vi "Amira Bladder Calibration V0.1.vi"() -> ()   [LabVIEW 2020]
uses:
  <userlib>/KQD LabVIEW User/Serial/Controls/SERIAL PortConfig.ctl
  <userlib>/KQD LabVIEW User/Serial/Controls/SERIAL BaudRate.ctl
  <userlib>/Amira UART/Public/TypeDefs/AUART StepDir.ctl
  <vilib>/Utility/file.llb/Write Delimited Spreadsheet (string).vi
  <userlib>/Amira UART/Amira UART.lvclass
  <userlib>/KQD LabVIEW User/Serial/Serial.lvlib
panel:
  out "Data":dbl[][](graph)
  in  "Iteration":i32
  in  "RunWith":cluster{"Steps":i32, "Rates":i32}={"Steps"=400, "Rates"=40}
  in  "Folder":path=path "C:/Amira Data/Strip"
  in  "StartAt":cluster{"Steps":i32, "Rates":i32}={"Steps"=950, "Rates"=200}
  out "Position":dbl[](graph)
  in  "DAQ":tag="Dev1/port0"
  out "UART":string
  in  "ComPort":refnum<visa-resource-name>
  in  "Config":T1={"BaudRate"=enum."460800", "StopBits"=10, "DataBits"=8, "Parity"=enum."None", "FlowControl"=2, "TimeOut"=1000, "TermChar"=10, "ReadTermEn"=TRUE} {"TermChar" format="%.0x"; "FlowControl" items=["None", "XON/XOFF", "RTS/CTS", "XON/XOFF & RTS/CTS", "DTR/DSR", "XON/XOFF & DTR/DSR"]; "DataBits" min=5 max=8 step=1; "StopBits" items=["1.0"=10, "1.5"=15, "2.0"=20]}
  out "ErrOut":errorcluster
  in  "ErrIn":errorcluster
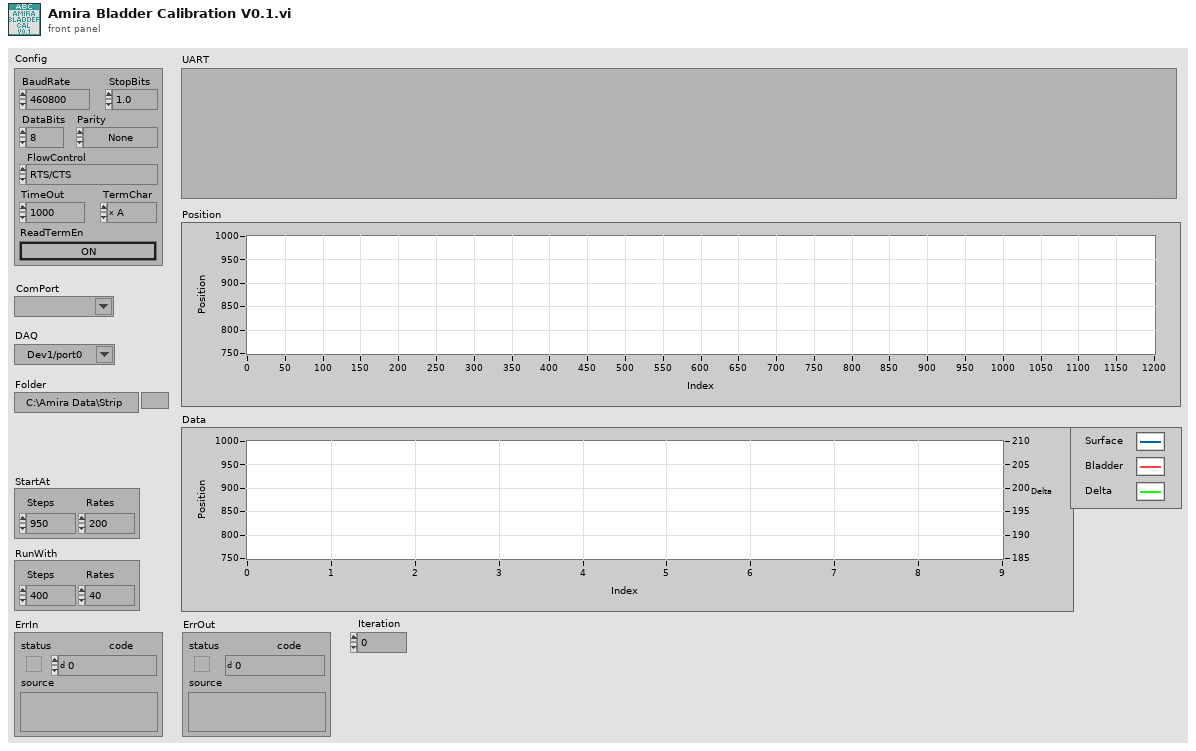
[diagram p1: front panel]
types:
  T1 = typedef "Serial.lvlib/SERIAL PortConfig.ctl" = cluster{"BaudRate":T2, "StopBits":u16, "DataBits":u16, "Parity":enum16{"None", "Odd", "Even", "Mark", "Space"}, "FlowControl":u16, "TimeOut":u32, "TermChar":u8, "ReadTermEn":bool}
  T2 = typedef "SERIAL BaudRate.ctl" = enum16{"2400", "4800", "7200", "9600", "14400", "19200", "28800", "38400", "57600", "115200", "128000", "230400", "460800", "921600"}
  T3 = typedef "Amira UART.lvclass/AUART StepDir.ctl" = enum16{"", "compress", "decompress"}
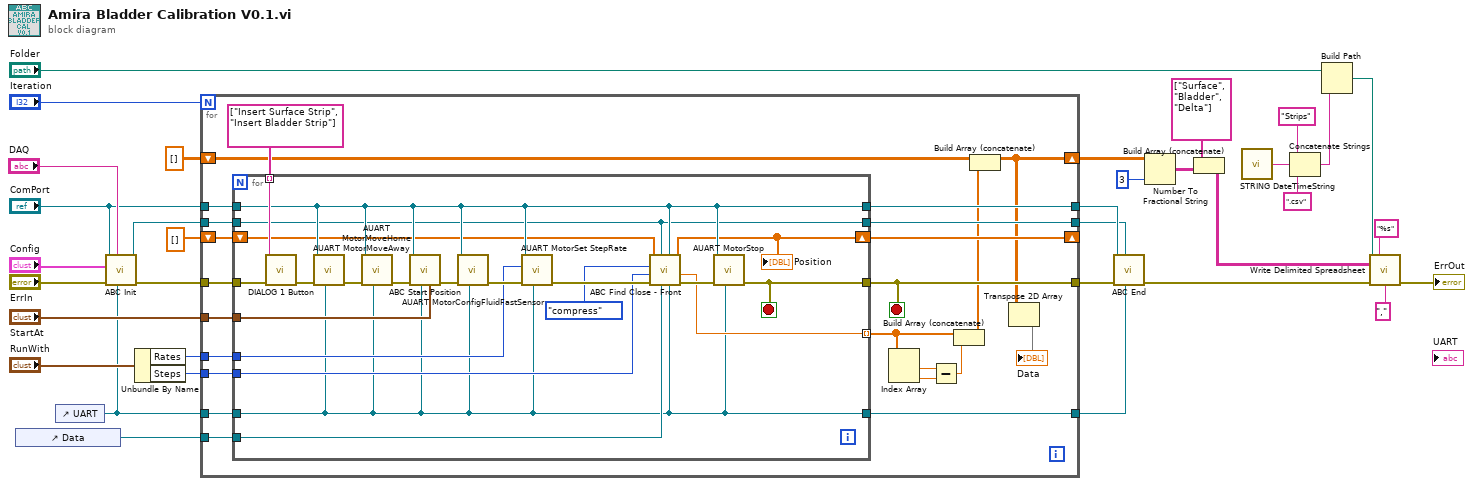
[diagram p0: block diagram]
diagram:
  n1 = control-ref of="Data"() -> (w29:refnum<vi>)
  n2 = control-ref of="UART"() -> (w24:refnum<vi>)
  n3 = call "ABC Init.vi"("UART"=w24, "DAQ"="DAQ", "ErrIn"="ErrIn", "PortConfig"="Config", "ComPort"="ComPort") -> ("ErrOut"=w25:errorcluster, "DaqTask"=w30:refnum<k21>)  [unwired: 5 in]
  n4 = Unbundle By Name("RunWith") -> ("Rates"=w27:i32, "Steps"=w26:i32)
  n5 = for {
    N: "Iteration" -> [_]
    tunnel: "StartAt" -> [w57]
    tunnel: w29 -> [w55]
    tunnel: w27 -> [w54]
    tunnel: w26 -> [w53]
    tunnel: "ComPort" -> [w50]
    tunnel: [w48] -> w21
    tunnel: w30 -> [w56]
    tunnel: [w47] -> w20
    tunnel: w25 -> [w52]
    tunnel: [w43] -> w22
    tunnel: w24 -> [w51]
    tunnel: [w45] -> w18
    shift-right: [w44] -> _
    shift-left: dbl[] [] ("DataOut") -> [w46]
    shift-right: [w37] -> w13
    shift-left: dbl[][] [] -> [w36]
    stop <- w43 stop-if-true
    n6 = for {
      tunnel: w57 -> [w74]
      tunnel: w56 -> [w62]
      tunnel: w55 -> [w72]
      tunnel: w54 -> [w70]
      tunnel: w53 -> [w69]
      tunnel: w51 -> [w58]
      tunnel: w50 -> [w63]
      tunnel: w52 -> [w68]
      tunnel: [w64] -> w43
      tunnel: string[] ["Insert Surface Strip", "Insert Bladder Strip"] -> [w65] mode=indexing
      tunnel: [w63] -> w48
      tunnel: [w62] -> w47
      shift-right: [w61] -> w44
      shift-left: w46 -> [w60]
      tunnel: [w59] -> w42 mode=indexing
      tunnel: [w58] -> w45
      stop <- w64 stop-if-true
      n7 = call <userlib>:"DIALOG 1 Button.vi"("ErrIn"=w68, "Msg"=w65) -> ("ErrOut"=w66:errorcluster)  [unwired: 9 in]
      n8 = call <userlib>:"AUART MotorMoveAway.vi"("UART"=w58, "ErrIn"=w66, "Port"=w63) -> ("ErrOut"=w67:errorcluster)  [unwired: 8 in]
      n9 = call <userlib>:"AUART MotorMoveHome.vi"("UART"=w58, "ErrIn"=w67, "Port"=w63) -> ("ErrOut"=w76:errorcluster)  [unwired: 7 in, 1 out]
      n10 = call "ABC Start Position.vi"("Start"=w74, "UART"=w58, "ErrIn"=w76, "ComPort"=w63) -> ("ErrOut"=w75:errorcluster)  [unwired: 6 in, 1 out]
      n11 = call <userlib>:"AUART MotorConfigFluidFastSensor.vi"("UART"=w58, "ErrIn"=w75, "Port"=w63) -> ("ErrOut"=w78:errorcluster)  [unwired: 8 in]
      n12 = call <userlib>:"AUART MotorSet StepRate.vi"("UART"=w58, "ErrIn"=w78, "step_rate"=w70, "Port"=w63) -> ("ErrOut"=w77:errorcluster)  [unwired: 7 in]
      n13 = call "ABC Find Close - Front.vi"("UART"=w58, "ComPort"=w63, "Data"=w72, "DaqTask"=w62, "ErrIn"=w77, "#Step"=w69, "Dir"=AUART_StepDir."compress" ("step_dir"), "DataIn"=w60) -> ("ErrOut"=w73:errorcluster, "FrontClose"=w59:dbl, "DataOut"=w61:dbl[])  [unwired: 1 in]
      "Position" <- w61
      n14 = call <userlib>:"AUART MotorStop.vi"("UART"=w58, "ErrIn"=w73, "Port"=w63) -> ("ErrOut"=w64:errorcluster)  [unwired: 8 in]
    }
    n15 = Index Array(array=w42) -> (element #1=w41:dbl, element #2=w40:dbl)  [unwired: 2 in]
    n16 = Subtract(x=w41, y=w40) -> (x-y=w39:dbl)
    n17 = Build Array (concatenate)(w42, w39) -> (w38:dbl[])
    n18 = Build Array (concatenate)(w36, w38) -> (w37:dbl[][])
    n19 = Transpose 2D Array(2D array=w37) -> (transposed array=→"Data":dbl[][])
  }
  n20 = call "ABC End.vi"("UART"=w18, "DaqTask"=w20, "ErrIn"=w22, "ComPort"=w21) -> ("ErrOut"=w15:errorcluster)  [unwired: 7 in]
  n21 = Number To Fractional String(number=w13, precision (6)=i16 3) -> (F-format string=w11:string[][])  [unwired: 2 in]
  n22 = Build Array (concatenate)(string[] ["Surface", "Bladder", "Delta"], w11) -> (w9:string[][])
  n23 = call <userlib>:"STRING DateTimeString.vi"() -> ("DateTimeStr"=w5:string)  [unwired: 2 in]
  n24 = Concatenate Strings("Strips" ("string"), w5, ".csv" ("string")) -> (w3:string)
  n25 = Build Path(base path="Folder", name or relative path=w3) -> (appended path=w2:path)
  n26 = call-poly <vilib>:"Write Delimited Spreadsheet.vi"("file path (dialog if empty)"=w2, "format (%s)"="%s", "2D data"=w9, "error in (no error)"=w15, "delimiter (\\t)"="," ("delimiter (\\t)")) -> ("error out"=→"ErrOut":errorcluster)  [unwired: 9 in, 1 out]
